vi "Motelist.vi"() -> (0 "error out":errorcluster, 2 "ComsInfo":cluster{"Name":string, "Com":string}[](array[cluster]))   [LabVIEW 2011]
panel:
  out "array":dbl[][](array[numeric])
  out "standard error":string
  out "standard output 2":string
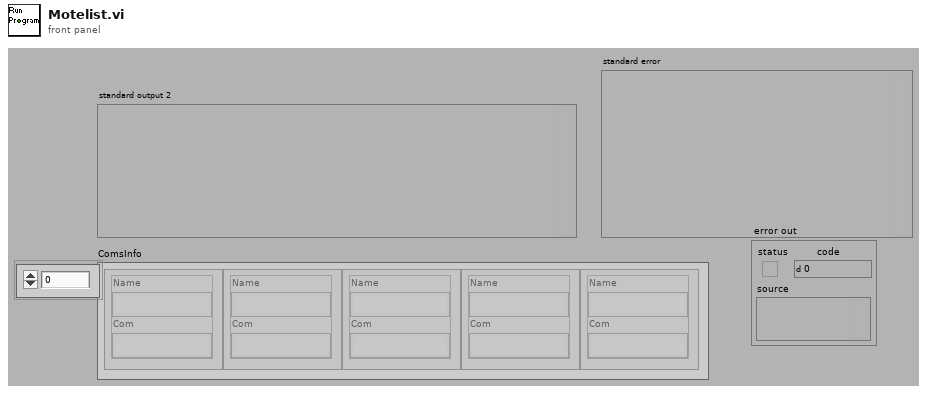
[diagram p1: front panel]
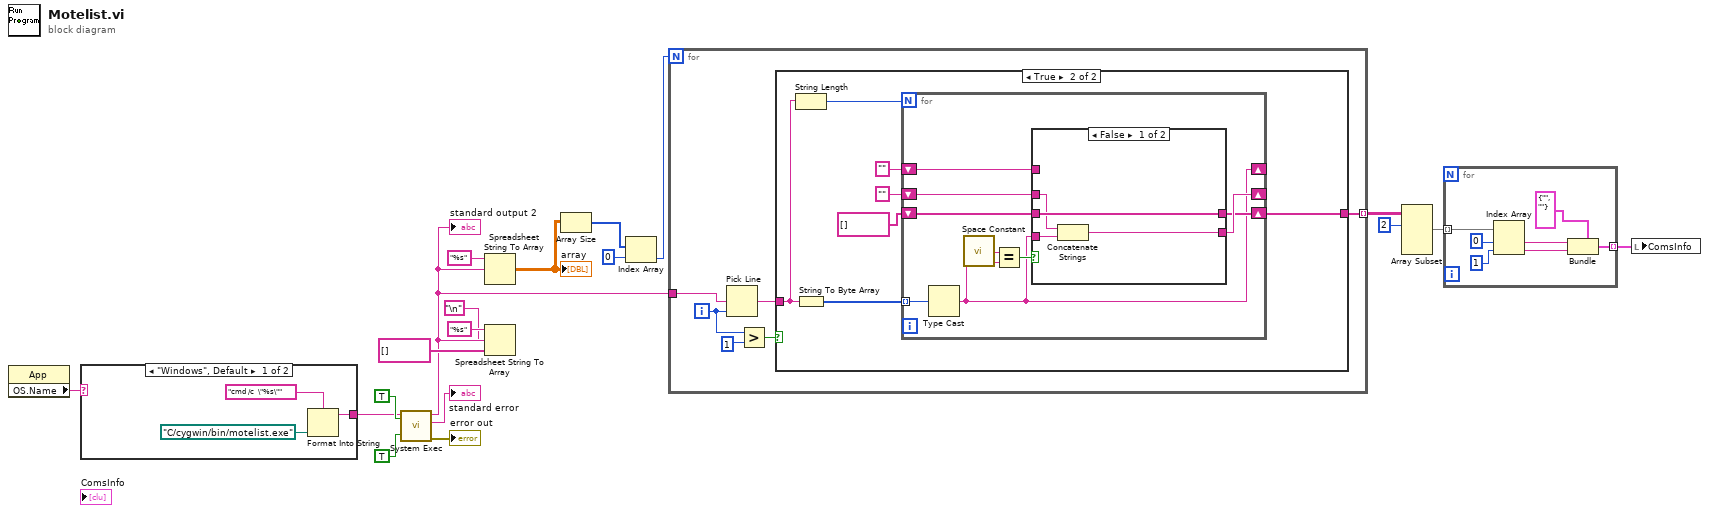
[diagram p0: block diagram]
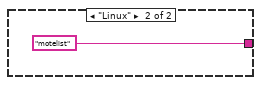
[diagram p2: hidden frame]
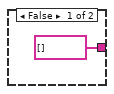
[diagram p3: hidden frame]
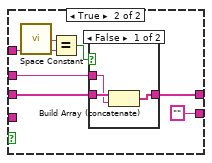
[diagram p4: hidden frame]
diagram:
  n1 = property class="App"() -> ("OS.Name"=w2:string)  [unwired: 2 in, 2 out]
  n2 = case shown="\"Windows\", Default" w2 {
    tunnel: [w20 "motelist"] -> w1
    frame "Windows", Default {
      n3 = Format Into String(format string="cmd /c  \"%s\"", path "C:/cygwin/bin/motelist.exe" ("input 1")) -> (resulting string=w20:string)  [unwired: 2 in, 1 out]
    }
    frame "Linux" {
    }
  }
  n4 = call <vilib>:"System Exec.vi"("run minimized? (F)"=TRUE, "wait until completion? (T)"=TRUE ("Wait until done"), "command line"=w1) -> ("error out"=→"error out":errorcluster, "standard error"=→"standard error":string, "standard output"=w10:string)  [unwired: 5 in, 1 out]
  "standard output 2" <- w10
  n5 = Spreadsheet String To Array(format string="%s", spreadsheet string=w10) -> (array=w15:dbl[][])  [unwired: 2 in]
  "array" <- w15
  n6 = Spreadsheet String To Array(delimiter (Tab)="\n", format string="%s", spreadsheet string=w10, array type (2D Dbl)=string[] []) -> ()  [unwired: 1 out]
  n7 = Array Size(array=w15) -> (size(s)=w14:i32[])
  n8 = Index Array(array=w14, index=0) -> (element=w12:i32)
  n9 = for {
    N: w12 -> [_]
    tunnel: w10 -> [w29]
    tunnel: [w24] -> w4 mode=indexing
    i -> [w27]
    n10 = Pick Line(multi-line string=w29, line index=w27) -> (output string=w25:string)  [unwired: 1 in]
    n11 = Greater?(x=w27, y=1) -> (0:w28:bool)
    n12 = case shown="True" w28 {
      tunnel: w25 -> [_ w36]
      tunnel: [string[] [] w32] -> w24
      frame False {
      }
      frame True {
        n13 = String Length(string=w36) -> (length=w37:i32)
        n14 = String To Byte Array(string=w36) -> (unsigned byte array=w35:u8[])
        n15 = for {
          N: w37 -> [_]
          tunnel: w35 -> [w45] mode=indexing
          shift-right: [w43] -> _
          shift-left: "" -> [w39]
          shift-right: [w42] -> w32
          shift-left: string[] [] -> [w41]
          shift-right: [w38] -> _
          shift-left: "" -> [w40]
          n16 = Type Cast(x=w45) -> (*(type *) &x=w38:string)  [unwired: 1 in]
          n17 = call <vilib>:"Space Constant.vi"() -> ("String"=w46:string)
          n18 = Equal?(x=w46, y=w38) -> (x = y?=w44:bool)
          n19 = case shown="False" w44 {
            tunnel: [w50 ""] -> w43
            tunnel: [w49 w54] -> w42
            tunnel: w41 -> [w49 w55]
            tunnel: w40 -> [_ w53]
            tunnel: w39 -> [w48 w51]
            tunnel: w38 -> [w47 _]
            frame False {
              n20 = Concatenate Strings(w48, w47) -> (w50:string)
            }
            frame True {
              n21 = call <vilib>:"Space Constant.vi"() -> ("String"=w52:string)
              n22 = Equal?(x=w52, y=w53) -> (x = y?=w56:bool)
              n23 = case shown="False" w56 {
                tunnel: w55 -> [w60 w61]
                tunnel: [w59 w61] -> w54
                tunnel: w51 -> [w58 _]
                frame False {
                  n24 = Build Array (concatenate)(w60, w58) -> (w59:string[])
                }
                frame True {
                }
              }
            }
          }
        }
      }
    }
  }
  n25 = Array Subset(array=w4, index (row)=2 ("index")) -> (w5:string[][])  [unwired: 3 in]
  n26 = for {
    tunnel: w5 -> [w68] mode=indexing
    tunnel: [w64] -> w7 mode=indexing
    n27 = Index Array(array=w68, index #1=0 ("index"), index #2=1 ("index")) -> (element #1=w63:string, element #2=w62:string)
    n28 = Bundle(cluster=cluster{string, string} {"", ""}, w63, w62) -> (w64:cluster{string, string})
  }
  n29 = local write "ComsInfo"(w7) -> ()
